vi "2 RudderControlPI.vi"(9 "use PID?":bool=TRUE, 10 "Desired Heading":dbl) -> (2 "Rudder Output":dbl)   [LabVIEW 2011]
uses:
  2 Typedefs/PI Constants.ctl
  2 Globals/2 Global.vi
  2 Globals/2 TuningConstants.vi
  <vilib>/addons/control/pid/NI_PID_pid.lvlib
  <vilib>/addons/control/pid/pid.llb/PID (DBL).vi
  <vilib>/ptbypt/NI_PtbyPt.lvlib
  <vilib>/addons/control/pid/NI_PID_autopid.lvlib
panel:
  out "Boolean 2":bool
  out "Boolean":bool
  out "PID gains out":T1={"proportional gain (Kc)"=1.0, "integral time (Ti, min)"=0.01, "derivative time (Td, min)"=0.0} {"derivative time (Td, min)" format="%.3f"; "integral time (Ti, min)" format="%.3f"; "proportional gain (Kc)" format="%.3f"}
  out "tuning completed?":bool
  in  "autotuning parameters":T2={"controller type"=1, "relay cycles"=3, "relay amplitude"=1.0, "control specification"=2, "PV noise level"=0.1} {"PV noise level" format="%.2f"; "control specification" items=["normal", "fast", "slow"]; "relay amplitude" format="%.2f"; "controller type" items=["PID", "PI", "P"]}
  in  "autotune? (F)":bool
  out "PID State":dbl format="%0.2f"
  out "PID setpoint":dbl
  out "PI Constants":T3={"Proportional Gain"=5000.0, "Integral Time"=0.2, "Derivative Time"=0.1}
  in  "Maximum Rudder":dbl=40.0
  out "Current Heading":dbl
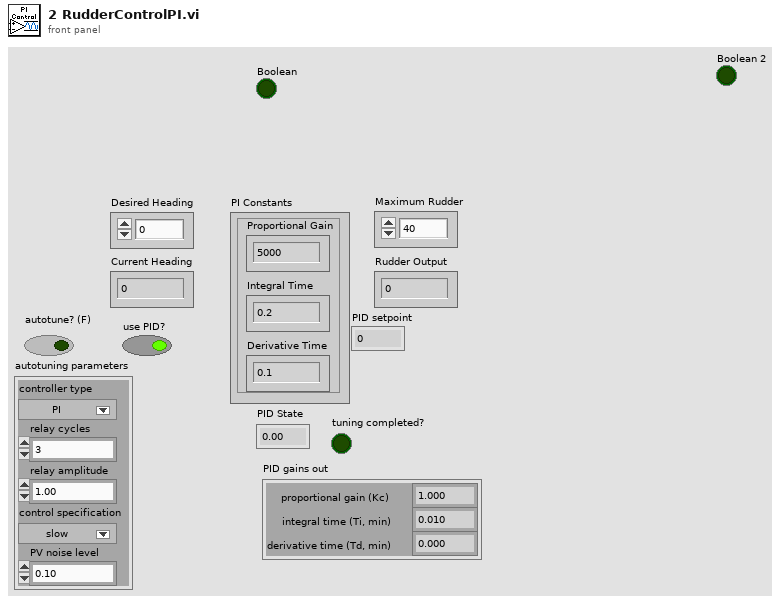
[diagram p1: front panel]
types:
  T1 = cluster{"proportional gain (Kc)":dbl, "integral time (Ti, min)":dbl, "derivative time (Td, min)":dbl}
  T2 = cluster{"controller type":u16, "relay cycles":i32, "relay amplitude":dbl, "control specification":u16, "PV noise level":dbl}
  T3 = typedef "PI Constants.ctl" = cluster{"Proportional Gain":dbl, "Integral Time":dbl, "Derivative Time":dbl}
  T4 = typedef "heading.ctl" = dbl
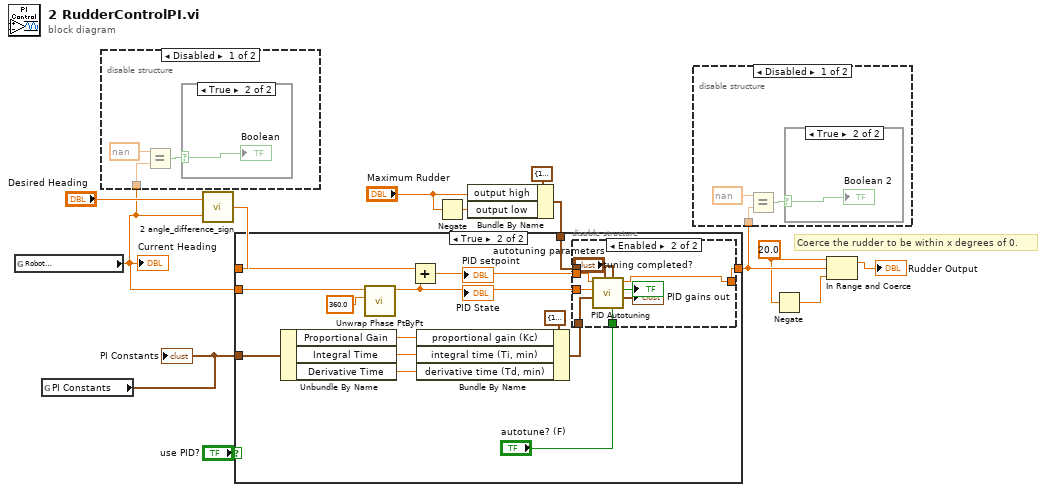
[diagram p0: block diagram]
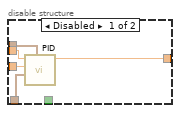
[diagram p7: hidden frame]
diagram:
  w1 = 20.0 ("upper limit")
  # "Coerce the rudder to be within x degrees of 0."
  n1 = global read "2 Global.vi" "Robot\nHeading"() -> (w5:T4)
  "Current Heading" <- w5
  n2 = global read "2 TuningConstants.vi" "PI Constants"() -> (w7:T3)
  "PI Constants" <- w7
  n3 = disable-structure shown="Disabled" {
    disable-tunnel: w5 -> [w16 _]
    frame Disabled {
      n4 = Equal?(x=nan, y=w16) -> (x = y?=w14:bool)
      n5 = case shown="True" w14 {
        selector: w14 -> [_ w17]
        frame False {
        }
        frame True {
          "Boolean" <- w17
        }
      }
    }
    frame Enabled {
    }
  }
  n6 = call "2 angle_difference_sign.vi"("Angle 2"=w5, "Angle 1"="Desired Heading") -> ("Difference"=w13:dbl)
  n7 = Negate(x="Maximum Rudder") -> (-x=w11:dbl)
  n8 = Bundle By Name(cluster=cluster{"output high":dbl, "output low":dbl} {"output high"=100.0, "output low"=-100.0} ("output range"), "output high"="Maximum Rudder", "output low"=w11) -> (w8:cluster{"output high":dbl, "output low":dbl})
  n9 = case shown="True" "use PID?" {
    tunnel: w13 -> [w18 w23]
    tunnel: w7 -> [_ w30]
    tunnel: w8 -> [_ w32]
    tunnel: w5 -> [_ w24]
    tunnel: [w18 w20] -> w4
    frame False {
    }
    frame True {
      n10 = Unbundle By Name(w30) -> ("Proportional Gain"=w28:dbl, "Integral Time"=w27:dbl, "Derivative Time"=w26:dbl)
      n11 = call <vilib>:"Unwrap Phase PtByPt.vi"("wrap base"=360.0, "phase"=w24) -> ("unwrapped phase"=w22:dbl)  [unwired: 9 in]
      "PID State" <- w22
      n12 = Add(x=w23, y=w22) -> (x+y=w21:dbl)
      "PID setpoint" <- w21
      n13 = Bundle By Name(cluster=T1 {"proportional gain (Kc)"=1.0, "integral time (Ti, min)"=0.01, "derivative time (Td, min)"=0.0} ("PID gains"), "proportional gain (Kc)"=w28, "integral time (Ti, min)"=w27, "derivative time (Td, min)"=w26) -> (w29:T1)
      n14 = disable-structure shown="Enabled" {
        disable-tunnel: w32 -> [w37 w42]
        disable-tunnel: w29 -> [w36 w44]
        disable-tunnel: w22 -> [w35 w45]
        disable-tunnel: w21 -> [w34 w46]
        disable-tunnel: [w33 w38] -> w20
        disable-tunnel: "autotune? (F)" -> [_ w43]
        frame Disabled {
          n15 = call-poly <vilib>:"PID.vi"("output range"=w37, "PID gains"=w36, "process variable"=w35, "setpoint"=w34) -> ("output"=w33:dbl)  [unwired: 6 in, 1 out]
        }
        frame Enabled {
          n16 = call <vilib>:"PID Autotuning.vi"("autotune? (F)"=w43, "autotuning parameters"="autotuning parameters", "output range"=w42, "PID gains"=w44, "process variable"=w45, "setpoint"=w46) -> ("PID gains out"=→"PID gains out":T1, "tuning completed?"=→"tuning completed?":bool, "output"=w38:dbl)  [unwired: 2 in, 1 out]
        }
      }
    }
  }
  n17 = disable-structure shown="Disabled" {
    disable-tunnel: w4 -> [w47 _]
    frame Disabled {
      n18 = Equal?(x=nan, y=w47) -> (x = y?=w49:bool)
      n19 = case shown="True" w49 {
        selector: w49 -> [_ w50]
        frame False {
        }
        frame True {
          "Boolean 2" <- w50
        }
      }
    }
    frame Enabled {
    }
  }
  n20 = Negate(x=w1) -> (-x=w2:dbl)
  n21 = In Range and Coerce(upper limit=w1, x=w4, lower limit=w2) -> (coerced(x)=→"Rudder Output":dbl)  [unwired: 1 out]
